vi "Waveform Channel Level.vi"(8 "error in (no error)":errorcluster, 11 "Node Ptr":T1 format="%.0x") -> (0 "error out":errorcluster)   [LabVIEW 2024, in "Embedded TDMS Logger System Explorer.lvlib"]
doc: "The waveform channel page for the UI to allow the user to configure the waveform channel, namely:\n- Decimation, desampling of the waveform\n- Name of the Waveform channel as logged in the TDMS file\n- Waveform channel being recorded\n- Meta Data to be tagged along the channel level in the TDMS file."
uses:
  Embedded TDMS Logger System Explorer.lvlib
  <vilib>/NI VeriStand/Custom Device API/Custom Device Item Ref.ctl
  <vilib>/NI VeriStand/Custom Device API/Get Item Property (Dependent Node Pointer).vi
  <vilib>/NI VeriStand/Custom Device API/Set Item Property (Dependent Node Pointer).vi
  <vilib>/NI VeriStand/Custom Device API/Get Item Property (I32).vi
  <vilib>/NI VeriStand/Custom Device API/Get Item Property (Variant).vi
  <vilib>/NI VeriStand/Custom Device API/Set Item Property (Variant).vi
  <vilib>/NI VeriStand/Custom Device API/Set Item Property (I32).vi
  NationalInstruments.VeriStand.SystemStorage
  <vilib>/NI VeriStand/Custom Device API/Custom Device API.lvlib
  <vilib>/NI VeriStand/Custom Device Tools/Custom Device Utility Library/Custom Device Utility Library.lvlib
  Shared/File Classes/Meta Data.ctl
panel:
  in  "Decimation":dbl
  in  "Channel":string(combo)
  in  "Group Level Meta Data":string[][](table)
  in  "Specific Header":cluster{"Section Name":string}={"Section Name"="Specific Page Settings"}
  in  "General Header":cluster{"Section Name":string}={"Section Name"="General Page Settings"}
  in  "Description":string
  in  "Channel Name":string
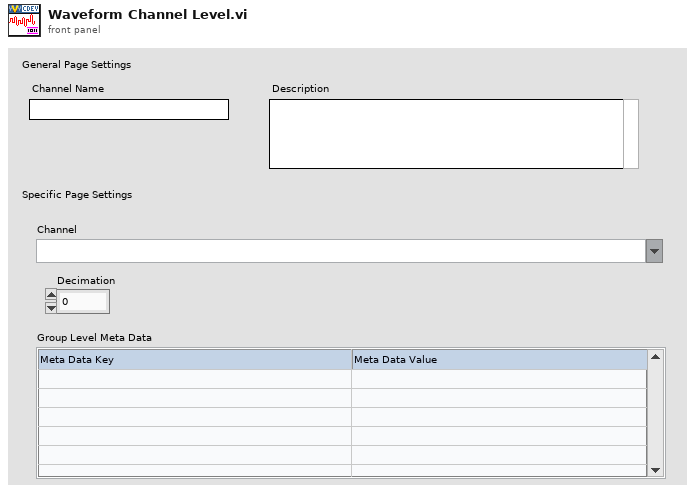
[diagram p1: front panel]
types:
  T1 = typedef "Custom Device API.lvlib/Custom Device Item Ref.ctl" = u64
  T2 = typedef "Meta Data.ctl" = cluster{"Key":string, "Value":string}
  T3 = typedef "Custom Device API.lvlib/Custom Device Pointer.ctl" = refnum<k24>
  T4 = typedef "Custom Device API.lvlib/Custom Device Item Info.ctl" = cluster{"Name":string, "Is Channel":bool, "GUID":string, "Is Waveform":bool}
  T5 = typedef "Custom Device API.lvlib/Custom Device Commands.ctl" = enum16{"Default", "Item renamed", "Shutdown", "Dynamic button pressed"}
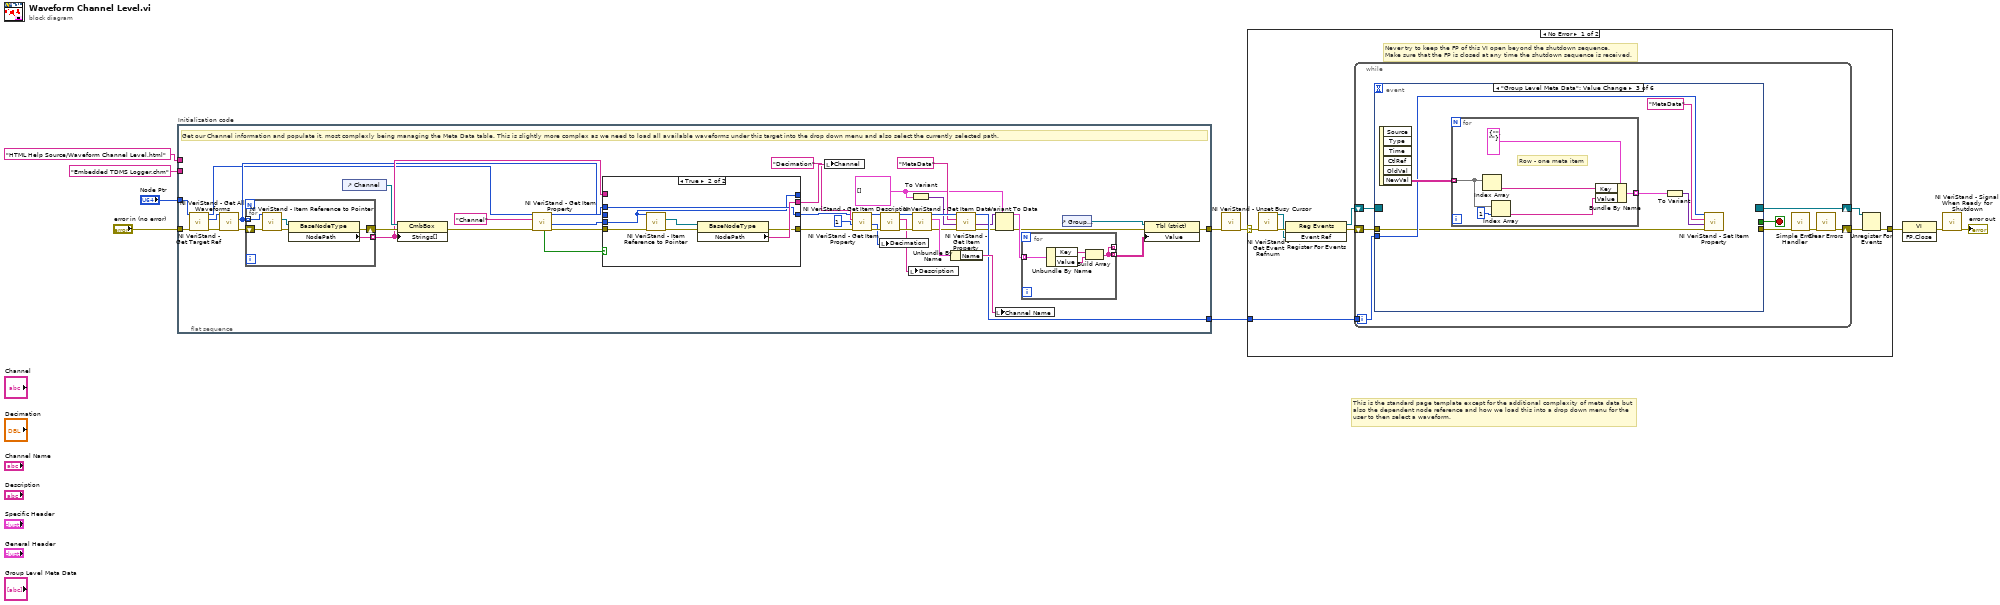
[diagram p0: block diagram]
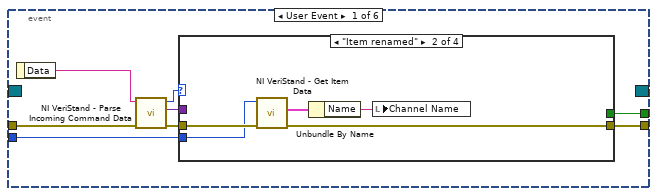
[diagram p2: hidden frame]
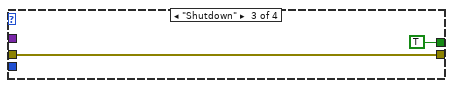
[diagram p4: hidden frame]
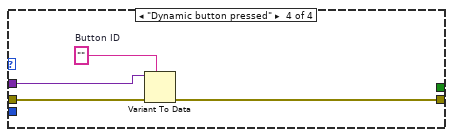
[diagram p5: hidden frame]
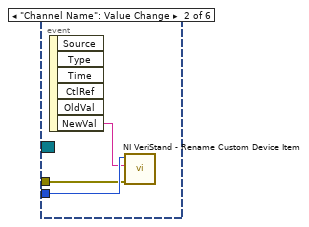
[diagram p6: hidden frame]
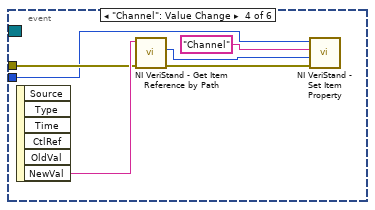
[diagram p7: hidden frame]
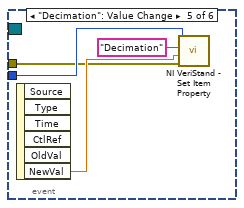
[diagram p8: hidden frame]
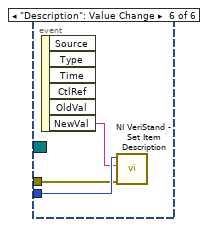
[diagram p9: hidden frame]
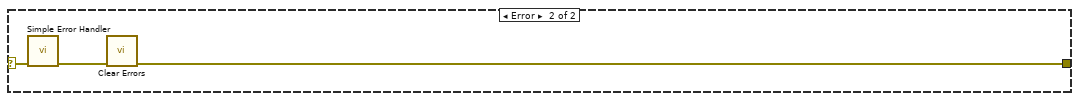
[diagram p10: hidden frame]
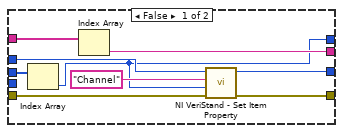
[diagram p11: hidden frame]
diagram:
  # "This is the standard page template except for the additional complexity of meta data but\nalso the dependent node reference and how we load this into a drop down menu for the\nuser to then select a waveform."
  n1 = flat-sequence "Initialization code" {
    tunnel: "error in (no error)" -> [w44]
    tunnel: "Node Ptr" -> [w43]
    tunnel: [w29] -> w6
    tunnel: [w38] -> w3
    tunnel: "HTML Help Source/Waveform Channel Level.html" ("CD_CHM_Section") -> [_]
    tunnel: "Embedded TDMS Logger.chm" ("CD_CHM_FileName") -> [_]
    frame #0 {
      w34 = T2[] []
      # "Get our Channel information and populate it, most complexly being managing the Meta Data table. This is slightly more complex as we need to load all available waveforms under this target into the drop down menu and also select the currently selected path."
      n2 = call <vilib>:"NI VeriStand - Get Target Ref.vi"("error in"=w44, "Item Ref in"=w43) -> ("error out"=w45:errorcluster, "Target Ref"=w18:T1, "Item Ref out"=w19:T1)  [unwired: 6 in, 1 out]
      n3 = call <vilib>:"NI VeriStand - Get All Waveforms.vi"("error in"=w45, "Section Ref in"=w18) -> ("error out"=w46:errorcluster, "Waveform Refs"=w20:T1[])  [unwired: 6 in, 2 out]
      n4 = for {
        tunnel: w20 -> [w78] mode=indexing
        shift-right: [w73] -> w42
        shift-left: w46 -> [w77]
        tunnel: [w74] -> w23 mode=indexing
        n5 = call <vilib>:"NI VeriStand - Item Reference to Pointer.vi"("error in (no error)"=w77, "Item Ref in"=w78) -> ("error out"=w76:errorcluster, "Node Pointer"=w75:T3)  [unwired: 6 in, 2 out]
        n6 = property class="BaseNodeType"(reference=w75, error in=w76) -> (error out=w73:errorcluster, "NodePath"=w74:string)  [unwired: 1 out]
      }
      n7 = control-ref of="Channel"() -> (w47:refnum<vi>)
      n8 = property class="CmbBox"(reference=w47, error in=w42, "Strings[]"=w23) -> (error out=w21:errorcluster)  [unwired: 1 out]
      n9 = call-poly <vilib>:"NI VeriStand - Get Item Property.vi"("error in (no error)"=w21, "Property Name"="Channel", "Item Ref in"=w19) -> ("error out"=w27:errorcluster, "Dependent Node Ref"=w26:T1, "Item Ref out"=w25:T1, "Found"=w24:bool)  [unwired: 5 in]
      n10 = case shown="True" w24 {
        tunnel: w26 -> [_ w63]
        tunnel: w27 -> [w59 w66]
        tunnel: [w57 w65] -> w22
        tunnel: w25 -> [w60 w64]
        tunnel: w23 -> [w58 _]
        tunnel: [w56 w64] -> w13
        tunnel: w20 -> [w55 _]
        tunnel: [w54 w62] -> w17
        tunnel: [w53 w63] -> _
        frame False {
          n11 = Index Array(array=w55) -> (element=w53:T1)  [unwired: 1 in]
          n12 = Index Array(array=w58) -> (element=w57:string)  [unwired: 1 in]
          n13 = call-poly <vilib>:"NI VeriStand - Set Item Property.vi"("error in (no error)"=w59, "Dependent Node Ref"=w53, "Property Name"="Channel", "Item Ref in"=w60) -> ("error out"=w54:errorcluster, "Item Ref out"=w56:T1)  [unwired: 5 in, 1 out]
        }
        frame True {
          n14 = call <vilib>:"NI VeriStand - Item Reference to Pointer.vi"("error in (no error)"=w66, "Item Ref in"=w63) -> ("error out"=w67:errorcluster, "Node Pointer"=w68:T3)  [unwired: 6 in, 2 out]
          n15 = property class="BaseNodeType"(reference=w68, error in=w67) -> (error out=w62:errorcluster, "NodePath"=w65:string)  [unwired: 1 out]
        }
      }
      n16 = local write "Channel"(w22) -> ()
      n17 = call-poly <vilib>:"NI VeriStand - Get Item Property.vi"("error in (no error)"=w17, "Default Value"=1, "Property Name"="Decimation", "Item Ref in"=w13) -> ("error out"=w16:errorcluster, "Value"=w11:i32, "Item Ref out"=w12:T1)  [unwired: 4 in, 1 out]
      n18 = local write "Decimation"(w11) -> ()
      n19 = call <vilib>:"NI VeriStand - Get Item Description.vi"("error in (no error)"=w16, "Item Ref in"=w12) -> ("error out"=w51:errorcluster, "Description"=w48:string, "Item Ref out"=w52:T1)  [unwired: 7 out]
      n20 = local write "Description"(w48) -> ()
      n21 = To Variant(anything=w34) -> (Variant=w37:variant)
      n22 = call <vilib>:"NI VeriStand - Get Item Data.vi"("error in (no error)"=w51, "Item Ref in"=w52) -> ("error out"=w41:errorcluster, "Item Info"=w50:T4, "Item Ref out"=w40:T1)  [unwired: 7 out]
      n23 = Unbundle By Name(w50) -> ("Name"=w49:string)
      n24 = call-poly <vilib>:"NI VeriStand - Get Item Property.vi"("error in (no error)"=w41, "Default Value"=w37, "Property Name"="MetaData", "Item Ref in"=w40) -> ("error out"=w36:errorcluster, "Value"=w35:variant, "Item Ref out"=w38:T1)  [unwired: 4 in, 1 out]
      n25 = Variant To Data(error in=w36, type=w34, Variant=w35) -> (data=w33:T2[], error out=w30:errorcluster)
      n26 = local write "Channel Name"(w49) -> ()
      n27 = for {
        tunnel: w33 -> [w72] mode=indexing
        tunnel: [w69] -> _ mode=indexing
        tunnel: [w69] -> w31 mode=indexing
        n28 = Unbundle By Name(w72) -> ("Key"=w71:string, "Value"=w70:string)
        n29 = Build Array(w71, w70) -> (w69:string[])
      }
      n30 = control-ref of="Group Level Meta Data"() -> (w32:refnum<vi>)
      n31 = property class="Tbl (strict)"(reference=w32, error in=w30, "Value"=w31) -> (error out=w29:errorcluster)  [unwired: 1 out]
    }
  }
  n32 = call <vilib>:"NI VeriStand - Unset Busy Cursor.vi"("error in (no error)"=w6) -> ("error out"=w5:errorcluster)  [unwired: 10 out]
  n33 = case shown="No Error" w5 {
    selector: w5 -> [w79 w146]
    tunnel: [w84 w144] -> w10
    tunnel: w3 -> [w80 _]
    frame No Error {
      # "Never try to keep the FP of this VI open beyond the shutdown sequence.\nMake sure that the FP is closed at any time the shutdown sequence is received."
      n34 = call <vilib>:"NI VeriStand - Get Event Refnum.vi"("error in (no error)"=w79) -> ("error out"=w87:errorcluster, "Event Ref"=w83:refnum<user-event>)  [unwired: 9 out]
      n35 = register-events(error in=w87, w83) -> (reference out=w81:refnum<event-registration>, error out=w82:errorcluster)  [unwired: 1 in]
      n36 = while {
        tunnel: w80 -> [w91]
        shift-right: [w88] -> w85
        shift-left: w82 -> [w94]
        shift-right: [w95] -> w86
        shift-left: w81 -> [w93]
        stop <- w92 stop-if-true
        n37 = event shown="[2] \"Group Level Meta Data\": Value Change" {
          selector: w93 -> [_ _ _ _ _ _]
          dyn-events: [_ _ _ _ _ _] -> w95
          timeout: _ -> [_ _ _ _ _ _]
          tunnel: w94 -> [w103 w116 w119 w133 w137 w142]
          tunnel: [w99 _ _ _ _ _] -> w92
          tunnel: [w98 _ _ _ _ _] -> w90
          tunnel: w91 -> [w97 w118 w120 w132 w138 w143]
          event User Event {
            n38 = event-data() -> ("Data"=w102:string)  [unwired: 1 out]
            n39 = call <vilib>:"NI VeriStand - Parse Incoming Command Data.vi"("error in (no error)"=w103, "Incoming data"=w102) -> ("error out"=w101:errorcluster, "Outgoing data"=w96:variant, "Action"=w100:T5)  [unwired: 7 out]
            n40 = case shown="\"Item renamed\"" w100 {
              tunnel: w101 -> [w104 w109 w110 w115]
              tunnel: [_ _ TRUE _] -> w99
              tunnel: [w104 w106 w110 w112] -> w98
              tunnel: w97 -> [_ w108 _ _]
              tunnel: w96 -> [_ _ _ w114]
              frame "Default", Default {
              }
              frame "Item renamed" {
                n41 = call <vilib>:"NI VeriStand - Get Item Data.vi"("error in (no error)"=w109, "Item Ref in"=w108) -> ("error out"=w106:errorcluster, "Item Info"=w107:T4)  [unwired: 8 out]
                n42 = Unbundle By Name(w107) -> ("Name"=w105:string)
                n43 = local write "Channel Name"(w105) -> ()
              }
              frame "Shutdown" {
              }
              frame "Dynamic button pressed" {
                w113 = ""  # Button ID
                n44 = Variant To Data(error in=w115, type=w113, Variant=w114) -> (error out=w112:errorcluster)  [unwired: 1 out]
              }
            }
          }
          event "Channel Name": Value Change {
            n45 = event-data() -> ("NewVal"=w117:string)  [unwired: 6 out]
            n46 = call <vilib>:"NI VeriStand - Rename Custom Device Item.vi"("error in (no error)"=w116, "New Name"=w117, "Item Ref in"=w118) -> ()  [unwired: 6 in, 3 out]
          }
          event "Group Level Meta Data": Value Change {
            n47 = event-data() -> ("NewVal"=w121:string[][])  [unwired: 6 out]
            n48 = for {
              tunnel: w121 -> [w129] mode=indexing
              tunnel: [w126] -> w124 mode=indexing
              # "Row - one meta item"
              n49 = Index Array(array=w129) -> (element=w127:string)  [unwired: 1 in]
              n50 = Index Array(array=w129, index=1) -> (element=w128:string)
              n51 = Bundle By Name(cluster=T2 {"Key"="", "Value"=""} ("Meta Data"), "Key"=w127, "Value"=w128) -> (w126:T2)
            }
            n52 = To Variant(anything=w124) -> (Variant=w123:variant)
            n53 = call-poly <vilib>:"NI VeriStand - Set Item Property.vi"("error in (no error)"=w119, "Value"=w123, "Property Name"="MetaData", "Item Ref in"=w120) -> ()  [unwired: 5 in, 3 out]
          }
          event "Channel": Value Change {
            n54 = event-data() -> ("NewVal"=w136:string)  [unwired: 6 out]
            n55 = call <vilib>:"NI VeriStand - Get Item Reference by Path.vi"("error in (no error)"=w133, "Item Path in"=w136) -> ("error out"=w134:errorcluster, "Item Ref"=w135:T1)  [unwired: 6 in, 2 out]
            n56 = call-poly <vilib>:"NI VeriStand - Set Item Property.vi"("error in (no error)"=w134, "Dependent Node Ref"=w135, "Property Name"="Channel", "Item Ref in"=w132) -> ()  [unwired: 5 in, 3 out]
          }
          event "Decimation": Value Change {
            n57 = event-data() -> ("NewVal"=w139:dbl)  [unwired: 6 out]
            n58 = call-poly <vilib>:"NI VeriStand - Set Item Property.vi"("error in (no error)"=w137, "Value"=w139, "Property Name"="Decimation", "Item Ref in"=w138) -> ()  [unwired: 5 in, 3 out]
          }
          event "Description": Value Change {
            n59 = event-data() -> ("NewVal"=w141:string)  [unwired: 6 out]
            n60 = call <vilib>:"NI VeriStand - Set Item Description.vi"("error in (no error)"=w142, "Description"=w141, "Item Ref in"=w143) -> ()  [unwired: 9 out]
          }
        }
        n61 = call <vilib>:"Simple Error Handler.vi"("error in (no error)"=w90) -> ("error out"=w89:errorcluster)  [unwired: 1 in, 7 out]
        n62 = call <vilib>:"Clear Errors.vi"("error in (no error)"=w89) -> ("error out"=w88:errorcluster)  [unwired: 1 in, 5 out]
      }
      n63 = Unregister For Events(event registration refnum=w86, error in=w85) -> (error out=w84:errorcluster)
    }
    frame Error {
      n64 = call <vilib>:"Simple Error Handler.vi"("error in (no error)"=w146) -> ("error out"=w145:errorcluster)  [unwired: 1 in, 7 out]
      n65 = call <vilib>:"Clear Errors.vi"("error in (no error)"=w145) -> ("error out"=w144:errorcluster)  [unwired: 1 in, 5 out]
    }
  }
  n66 = invoke class="VI" method="FP.Close"(error in=w10) -> (error out=w9:errorcluster)  [unwired: 2 in, 2 out]
  n67 = call <vilib>:"NI VeriStand - Signal When Ready for Shutdown.vi"("error in (no error)"=w9) -> ("error out"=→"error out":errorcluster)  [unwired: 10 out]
